vi "AddParamChannels_Create one Parameter per Discrete Bit.vi"(8 "error in (no error)":errorcluster, 11 "Parameters In":T1[](array[typedef])) -> (0 "error out":errorcluster, 3 "Parameters Out":T1[](array[typedef]))   [LabVIEW 2019, in "Ballard Arinc-429 System Explorer.lvlib"]
uses:
  Ballard Arinc-429 System Explorer.lvlib
  Parse Parameters File/XML_Parameter.ctl
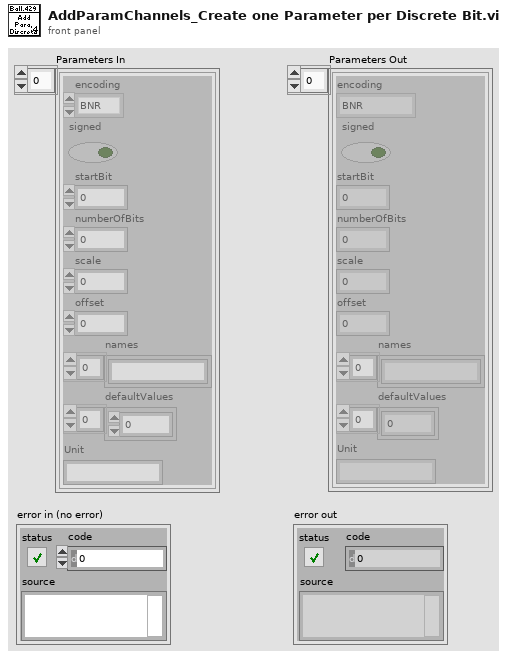
[diagram p1: front panel]
types:
  T1 = typedef "XML_Parameter.ctl" = cluster{"encoding":enum16{"BNR", "BCD", "Discrete"}, "signed":bool, "startBit":i32, "numberOfBits":i32, "scale":dbl, "offset":dbl, "names":string[], "defaultValues":dbl[], "Unit":string}
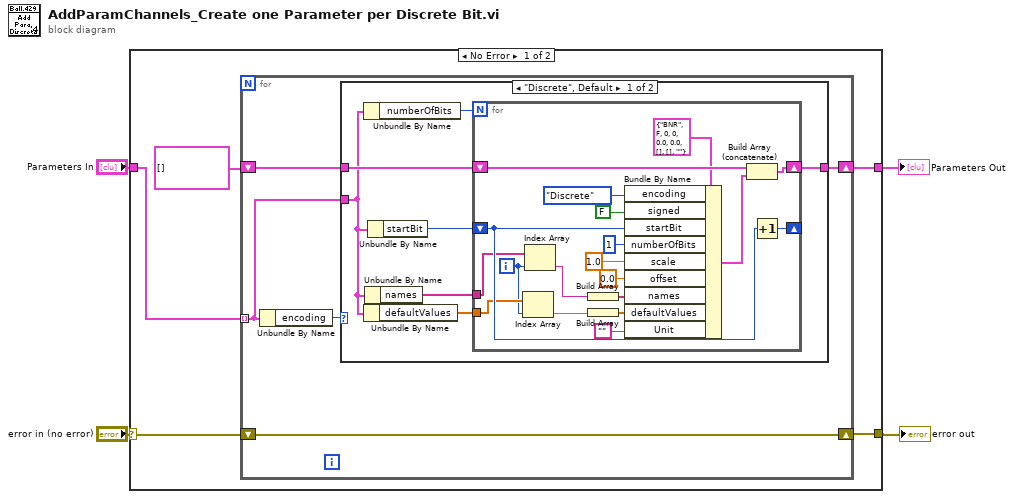
[diagram p0: block diagram]
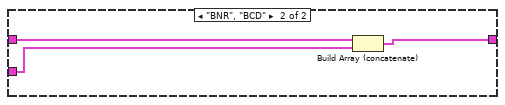
[diagram p2: hidden frame]
diagram:
  n1 = case shown="No Error" "error in (no error)" {
    selector: "error in (no error)" -> [w9 w45]
    tunnel: [w8 w45] -> w3
    tunnel: "Parameters In" -> [w7 w44]
    tunnel: [w6 w44] -> w1
    frame No Error {
      n2 = for {
        shift-right: [w11] -> w6
        shift-left: T1[] [] -> [w13]
        shift-right: [w10] -> w8
        shift-left: w9 -> [w10]
        tunnel: w7 -> [w12] mode=indexing
        n3 = Unbundle By Name(w12) -> ("encoding"=w14:enum16{"BNR", "BCD", "Discrete"})
        n4 = case shown="\"Discrete\", Default" w14 {
          tunnel: w13 -> [w20 w41]
          tunnel: w12 -> [w16 w43]
          tunnel: [w19 w42] -> w11
          frame "Discrete", Default {
            n5 = Unbundle By Name(w16) -> ("numberOfBits"=w21:i32)
            n6 = Unbundle By Name(w16) -> ("defaultValues"=w18:dbl[])
            n7 = Unbundle By Name(w16) -> ("names"=w17:string[])
            n8 = Unbundle By Name(w16) -> ("startBit"=w15:i32)
            n9 = for {
              N: w21 -> [_]
              shift-right: [w31] -> w19
              shift-left: w20 -> [w32]
              tunnel: w18 -> [w24]
              tunnel: w17 -> [w26]
              shift-right: [w27] -> _
              shift-left: w15 -> [w28]
              i -> [w23]
              n10 = Index Array(array=w24, index=w23) -> (element=w22:dbl)
              n11 = Index Array(array=w26, index=w23) -> (element=w25:string)
              n12 = Build Array(w25) -> (w40:string[])
              n13 = Build Array(w22) -> (w39:dbl[])
              n14 = Bundle By Name(cluster=T1 {"encoding"=enum."BNR", "signed"=FALSE, "startBit"=0, "numberOfBits"=0, "scale"=0.0, "offset"=0.0, "names"=[], "defaultValues"=[], "Unit"=""} ("Parameter"), "encoding"=enum16{"BNR", "BCD", "Discrete"}."Discrete", "signed"=FALSE, "startBit"=w28, "numberOfBits"=1, "scale"=1.0, "offset"=0.0, "names"=w40, "defaultValues"=w39, "Unit"="") -> (w30:T1)
              n15 = Build Array (concatenate)(w32, w30) -> (w31:T1[])
              n16 = Increment(x=w28) -> (x+1=w27:i32)
            }
          }
          frame "BNR", "BCD" {
            n17 = Build Array (concatenate)(w41, w43) -> (w42:T1[])
          }
        }
      }
    }
    frame Error {
    }
  }
  "Parameters Out" <- w1
  "error out" <- w3
